vi "VI2.vi"(1 "Cluster with a string inside it 2":cluster{"String inside a cluster":string}={"String inside a cluster"="123456"}, 9 "Cluster with a string inside it":cluster{"String inside a cluster":string}, 11 "Boolean input":bool) -> (3 "Boolean indicator.":bool)   [LabVIEW 2025]
panel:
  in  "Numeric":dbl
  in  "String":string
  out "Text  indicator":string
  in  "A text indicator":string
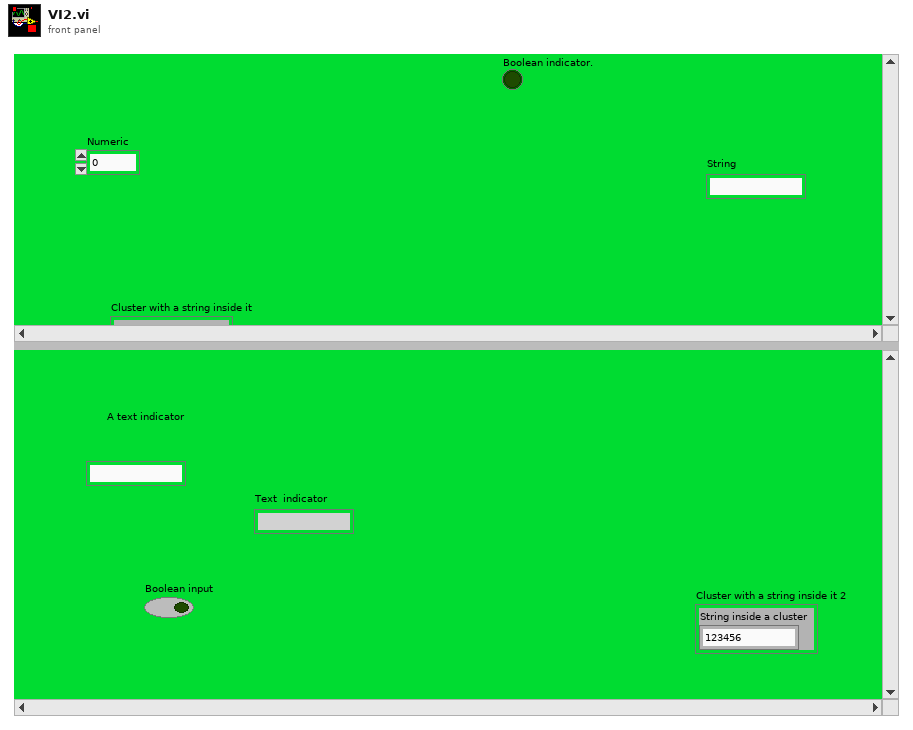
[diagram p1: front panel]
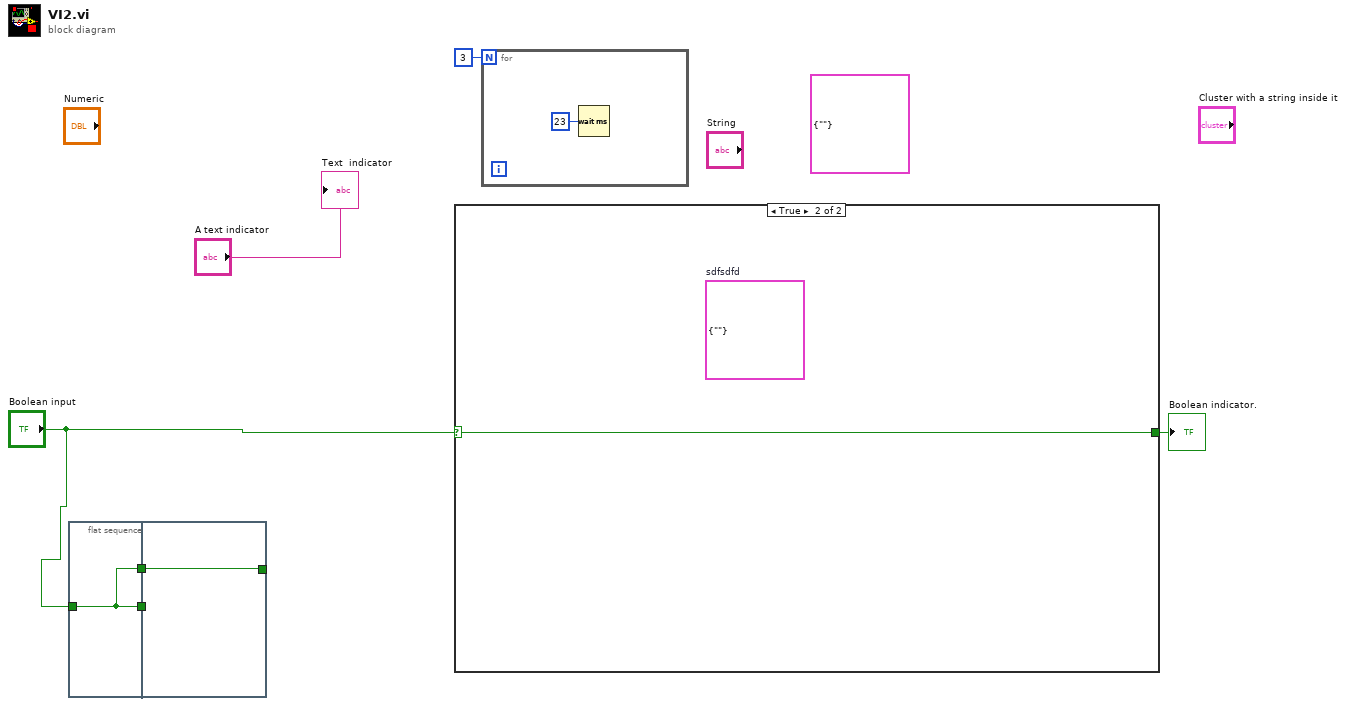
[diagram p0: block diagram]
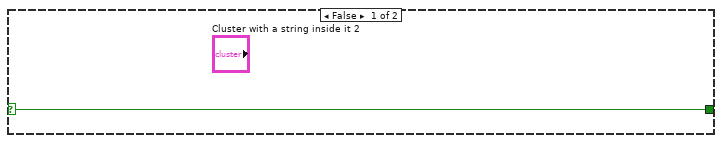
[diagram p2: hidden frame]
diagram:
  (unwired) cluster{string} {""}
  n1 = flat-sequence {
    tunnel: "Boolean input" -> [w7]
    tunnel: [w7] -> w2
    tunnel: [w7] -> w1
    tunnel: w2 -> [_]
    tunnel: w1 -> [w8]
    tunnel: [w8] -> _
    frame #0 {
    }
    frame #1 {
    }
  }
  n2 = case shown="True" "Boolean input" {
    selector: "Boolean input" -> [w9 w10]
    tunnel: [w9 w10] -> w6
    frame False {
    }
    frame True {
      (unwired) cluster{string} {""}  # sdfsdfd
    }
  }
  "Boolean indicator." <- w6
  n3 = for {
    N: 3 -> [_]
    n4 = Wait (ms)(milliseconds to wait=u32 23) -> ()  [unwired: 1 out]
  }
  "Text  indicator" <- "A text indicator"
